vi "SinCos.vi"(1 "SinCos3":refnum<class "SinCos3.lvclass">, 7 "X":sgl) -> (6 "sinX":sgl, 10 "cosX":sgl)   [LabVIEW 2017, in "SinCos3.lvclass"]
uses:
  SinCos3.lvclass
  <vilib>/rvi/FXPMathLib/FxpSinAndCos/subVIs/nifxpmath_SinAndCos_SimConfig.ctl
  <vilib>/rvi/FXPMathLib/FxpSinAndCos/simVIs/DllFxpSinAndCosTemp_sub.vi
  <vilib>/rvi/FXPMathLib/FxpSinAndCos/XNode/nifxpmath_SinAndCos.xnode
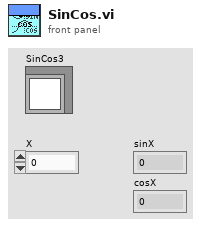
[diagram p1: front panel]
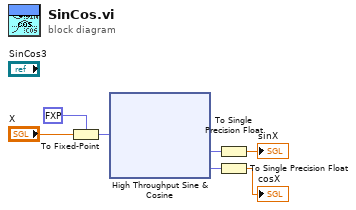
[diagram p0: block diagram]
diagram:
  n1 = To Fixed-Point(fixed-point type=fxp<+/-,16,1> 0.0 ("x (pi)"), number="X") -> (fixed-point=w4:fxp<+/-,16,1>)
  n2 = xnode "High Throughput Sine & Cosine"("x (pi)"=w4) -> ("sin(x)"=w1:fxp<+/-,16,2>, "cos(x)"=w2:fxp<+/-,16,2>)
  n3 = To Single Precision Float(number=w1) -> (single precision float=→"sinX":sgl)
  n4 = To Single Precision Float(number=w2) -> (single precision float=→"cosX":sgl)
